vi "M9700 Modbus Demo.vi"(0 "Serial Port:":refnum<visa-resource-name>="COM1", 1 "Voltage(V)":sgl=10.0 format="%#.5g", 2 "Current(A)":sgl=1.0 format="%#.5g", 3 "Resistance(Ohm)":sgl=100.0 format="%#.5g", 4 "Power(W)":sgl=30.0 format="%#.5g", 5 "error in (no error)":errorcluster, 6 "BaudRate:":u16(ring)=1 items=["  2400", "  9600", "  14400", "  28800", "  57600", "  115200"], 7 "Set Voltage":bool, 10 "Load Address":u8=1 min=1 max=200 format="%.0x", 11 "Set Current":bool, 12 "Input ON":bool, 13 "Set Resistance":bool, 14 "Input OFF":bool, 15 "Set Power":bool, 16 "Read Actual Value":bool, 17 "Exit":bool, 18 "Read Input State":bool) -> (19 "error out":errorcluster)   [LabVIEW 2014]
uses:
  M9700 Driver/86/vi.lib/M9700 Modbus.llb/CTL CMD Register.ctl
  M9700 Driver/85/vi.lib/M9700 Modbus.llb/CTL Register Address.ctl
  <vilib>/Instr/_visa.llb/VISA Configure Serial Port (Instr).vi
panel:
  in  "Configure Serial Port":bool
  in  "Short Mode":bool
  out "Actual Power(W)":sgl format="%#.5g"
  out "Actual Resistance(Ohm)":sgl format="%#.5g"
  out "Actual Current(A)":sgl format="%#.5g"
  out "Actual Voltage(V)":sgl format="%#.5g"
  out "Input State":bool
  in  "About":bool
  in  "Parity:":u16(ring) items=["  None", "  Odd", "  Even"]
  # "This example shows how communication is generated between M97 series electronic load \n and LabVIEW Program by M9700 MODBUS LabVIEW Driver. \n."
  # "Serial Port Parameter:"
  # "Work Mode:"
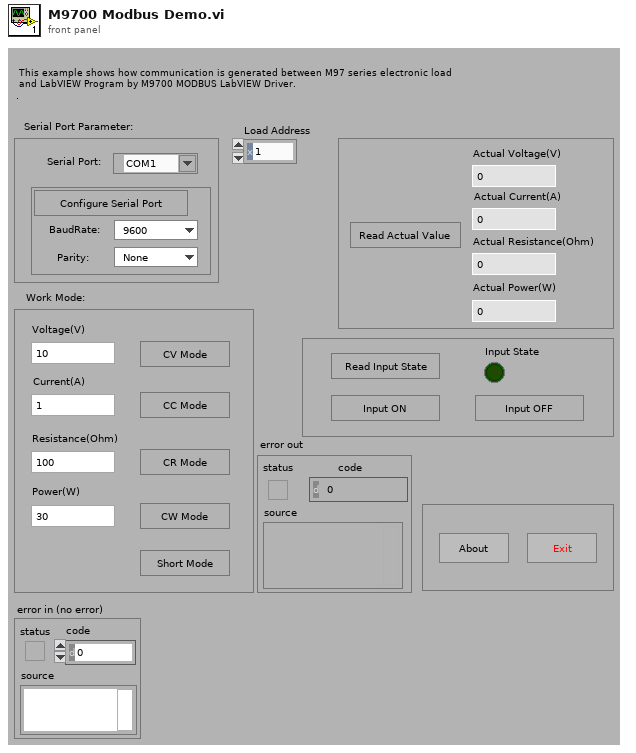
[diagram p1: front panel]
types:
  T1 = typedef "CTL CMD Register.ctl" = u8
  T2 = typedef "CTL Register Address.ctl" = u16
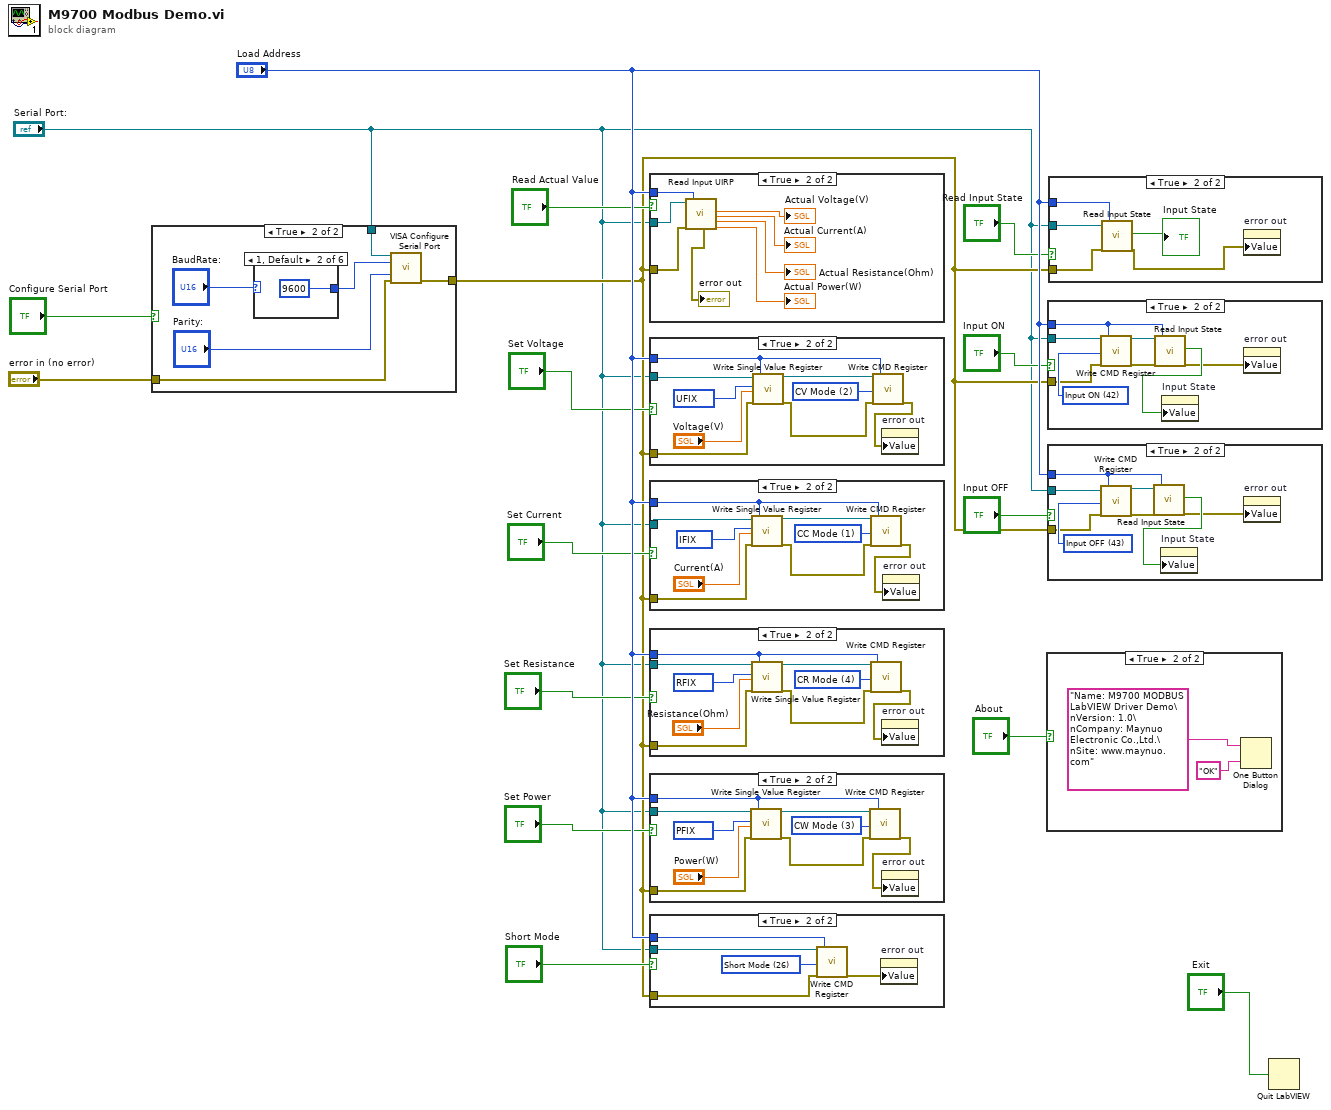
[diagram p0: block diagram]
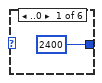
[diagram p3: hidden frame]
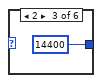
[diagram p4: hidden frame]
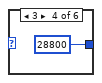
[diagram p5: hidden frame]
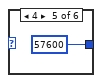
[diagram p6: hidden frame]
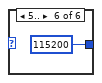
[diagram p7: hidden frame]
diagram:
  n1 = case shown="True" "Configure Serial Port" {
    tunnel: [w17 w23] -> w4
    tunnel: "Serial Port:" -> [_ w19]
    tunnel: "error in (no error)" -> [w17 w18]
    frame False {
    }
    frame True {
      n2 = case shown="1, Default" "BaudRate:" {
        tunnel: [2400 9600 14400 28800 57600 115200] -> w21
        frame ..0 {
        }
        frame 1, Default {
        }
        frame 2 {
        }
        frame 3 {
        }
        frame 4 {
        }
        frame 5.. {
        }
      }
      n3 = call-poly "VISA Configure Serial Port"("VISA resource name"=w19, "baud rate (9600)"=w21, "parity (0:none)"="Parity:", "error in (no error)"=w18) -> ("error out"=w23:errorcluster)  [unwired: 2 in, 9 out]
    }
  }
  n4 = case shown="True" "Read Actual Value" {
    tunnel: "Load Address" -> [_ w37]
    tunnel: "Serial Port:" -> [_ w36]
    tunnel: w4 -> [_ w31]
    frame False {
    }
    frame True {
      n5 = call "Read Input UIRP.vi"("VISA resource name"=w36, "error in"=w31, "Load Address"=w37) -> ("error out"=→"error out":errorcluster, "Actual Voltage(V)"=→"Actual Voltage(V)":sgl, "Actual Current(A)"=→"Actual Current(A)":sgl, "Actual Resistance(Ohm)"=→"Actual Resistance(Ohm)":sgl, "Actual Power(W)"=→"Actual Power(W)":sgl)  [unwired: 12 out]
    }
  }
  n6 = case shown="True" "Set Voltage" {
    tunnel: "Load Address" -> [_ w42]
    tunnel: "Serial Port:" -> [_ w46]
    tunnel: w4 -> [_ w40]
    frame False {
    }
    frame True {
      w41 = T1 2 items=["CC Mode"=1, "CV Mode"=2, "CW Mode"=3, "CR Mode"=4, "Short Mode"=26, "Set SysPara"=41, "Input ON"=42, "Input OFF"=43] ("CMD Register Value")
      w44 = T2 2563 items=["REMOTE"=1283, "ISTATE"=1296, "CMD"=2560, "IFIX"=2561, "UFIX"=2563, "PFIX"=2565, "RFIX"=2567, "IMAX"=2612, "UMAX"=2614, "PMAX"=2616, "U"=2816, "I"=2818, "MODEL"=2822, "EDITION"=2823] ("Register Address")
      n7 = call "Write Single Value Register.vi"("VISA resource name"=w46, "Starting Address(HEX)"=w44, "Register Single Value"="Voltage(V)", "error in"=w40, "Load Address"=w42) -> ("VISA resource name out"=w43:refnum<visa-resource-name>, "error out"=w39:errorcluster)  [unwired: 13 out]
      n8 = call "Write CMD Register.vi"("VISA resource name"=w43, "CMD Value"=w41, "error in"=w39, "Load Address"=w42) -> ("error out"=w38:errorcluster)  [unwired: 15 out]
      n9 = property on="error out" class="Clust (strict)"("Value"=w38) -> ()  [unwired: 2 in, 2 out]
    }
  }
  n10 = case shown="True" "Set Current" {
    tunnel: "Load Address" -> [_ w55]
    tunnel: "Serial Port:" -> [_ w51]
    tunnel: w4 -> [_ w49]
    frame False {
    }
    frame True {
      w52 = T1 1 items=["CC Mode"=1, "CV Mode"=2, "CW Mode"=3, "CR Mode"=4, "Short Mode"=26, "Set SysPara"=41, "Input ON"=42, "Input OFF"=43] ("CMD Register Value")
      w54 = T2 2561 items=["REMOTE"=1283, "ISTATE"=1296, "CMD"=2560, "IFIX"=2561, "UFIX"=2563, "PFIX"=2565, "RFIX"=2567, "IMAX"=2612, "UMAX"=2614, "PMAX"=2616, "U"=2816, "I"=2818, "MODEL"=2822, "EDITION"=2823] ("Register Address")
      n11 = call "Write Single Value Register.vi"("VISA resource name"=w51, "Starting Address(HEX)"=w54, "Register Single Value"="Current(A)", "error in"=w49, "Load Address"=w55) -> ("VISA resource name out"=w50:refnum<visa-resource-name>, "error out"=w48:errorcluster)  [unwired: 13 out]
      n12 = call "Write CMD Register.vi"("VISA resource name"=w50, "CMD Value"=w52, "error in"=w48, "Load Address"=w55) -> ("error out"=w47:errorcluster)  [unwired: 15 out]
      n13 = property on="error out" class="Clust (strict)"("Value"=w47) -> ()  [unwired: 2 in, 2 out]
    }
  }
  n14 = case shown="True" "Set Resistance" {
    tunnel: "Serial Port:" -> [_ w62]
    tunnel: "Load Address" -> [_ w64]
    tunnel: w4 -> [_ w58]
    frame False {
    }
    frame True {
      w59 = T1 4 items=["CC Mode"=1, "CV Mode"=2, "CW Mode"=3, "CR Mode"=4, "Short Mode"=26, "Set SysPara"=41, "Input ON"=42, "Input OFF"=43] ("CMD Register Value")
      w61 = T2 2567 items=["REMOTE"=1283, "ISTATE"=1296, "CMD"=2560, "IFIX"=2561, "UFIX"=2563, "PFIX"=2565, "RFIX"=2567, "IMAX"=2612, "UMAX"=2614, "PMAX"=2616, "U"=2816, "I"=2818, "MODEL"=2822, "EDITION"=2823] ("Register Address")
      n15 = call "Write Single Value Register.vi"("VISA resource name"=w62, "Starting Address(HEX)"=w61, "Register Single Value"="Resistance(Ohm)", "error in"=w58, "Load Address"=w64) -> ("VISA resource name out"=w63:refnum<visa-resource-name>, "error out"=w57:errorcluster)  [unwired: 13 out]
      n16 = call "Write CMD Register.vi"("VISA resource name"=w63, "CMD Value"=w59, "error in"=w57, "Load Address"=w64) -> ("error out"=w56:errorcluster)  [unwired: 15 out]
      n17 = property on="error out" class="Clust (strict)"("Value"=w56) -> ()  [unwired: 2 in, 2 out]
    }
  }
  n18 = case shown="True" "Set Power" {
    tunnel: "Serial Port:" -> [_ w73]
    tunnel: "Load Address" -> [_ w71]
    tunnel: w4 -> [_ w68]
    frame False {
    }
    frame True {
      w69 = T1 3 items=["CC Mode"=1, "CV Mode"=2, "CW Mode"=3, "CR Mode"=4, "Short Mode"=26, "Set SysPara"=41, "Input ON"=42, "Input OFF"=43] ("CMD Register Value")
      w70 = T2 2565 items=["REMOTE"=1283, "ISTATE"=1296, "CMD"=2560, "IFIX"=2561, "UFIX"=2563, "PFIX"=2565, "RFIX"=2567, "IMAX"=2612, "UMAX"=2614, "PMAX"=2616, "U"=2816, "I"=2818, "MODEL"=2822, "EDITION"=2823] ("Register Address")
      n19 = call "Write Single Value Register.vi"("VISA resource name"=w73, "Starting Address(HEX)"=w70, "Register Single Value"="Power(W)", "error in"=w68, "Load Address"=w71) -> ("VISA resource name out"=w72:refnum<visa-resource-name>, "error out"=w66:errorcluster)  [unwired: 13 out]
      n20 = call "Write CMD Register.vi"("VISA resource name"=w72, "CMD Value"=w69, "error in"=w66, "Load Address"=w71) -> ("error out"=w65:errorcluster)  [unwired: 15 out]
      n21 = property on="error out" class="Clust (strict)"("Value"=w65) -> ()  [unwired: 2 in, 2 out]
    }
  }
  n22 = case shown="True" "Short Mode" {
    tunnel: "Serial Port:" -> [_ w78]
    tunnel: "Load Address" -> [_ w76]
    tunnel: w4 -> [_ w75]
    frame False {
    }
    frame True {
      w77 = T1 26 items=["CC Mode"=1, "CV Mode"=2, "CW Mode"=3, "CR Mode"=4, "Short Mode"=26, "Set SysPara"=41, "Input ON"=42, "Input OFF"=43] ("CMD Register Value")
      n23 = call "Write CMD Register.vi"("VISA resource name"=w78, "CMD Value"=w77, "error in"=w75, "Load Address"=w76) -> ("error out"=w74:errorcluster)  [unwired: 15 out]
      n24 = property on="error out" class="Clust (strict)"("Value"=w74) -> ()  [unwired: 2 in, 2 out]
    }
  }
  n25 = case shown="True" "About" {
    frame False {
    }
    frame True {
      n26 = One Button Dialog(message="Name: M9700 MODBUS LabVIEW Driver Demo\nVersion: 1.0\nCompany: Maynuo Electronic Co.,Ltd.\nSite: www.maynuo.com", button name ("OK")="OK") -> ()  [unwired: 1 out]
    }
  }
  n27 = case shown="True" "Input ON" {
    tunnel: "Serial Port:" -> [_ w88]
    tunnel: "Load Address" -> [_ w84]
    tunnel: w4 -> [_ w83]
    frame False {
    }
    frame True {
      w87 = T1 42 items=["CC Mode"=1, "CV Mode"=2, "CW Mode"=3, "CR Mode"=4, "Short Mode"=26, "Set SysPara"=41, "Input ON"=42, "Input OFF"=43] ("CMD Register Value")
      n28 = call "Write CMD Register.vi"("VISA resource name"=w88, "CMD Value"=w87, "error in"=w83, "Load Address"=w84) -> ("VISA resource name out"=w86:refnum<visa-resource-name>, "error out"=w82:errorcluster)  [unwired: 14 out]
      n29 = call "Read Input State.vi"("VISA resource name"=w86, "error in"=w82, "Load Address"=w84) -> ("Input State(ON/OFF)"=w85:bool, "error out"=w81:errorcluster)  [unwired: 15 out]
      n30 = property on="Input State" class="Bool (strict)"("Value"=w85) -> ()  [unwired: 2 in, 2 out]
      n31 = property on="error out" class="Clust (strict)"("Value"=w81) -> ()  [unwired: 2 in, 2 out]
    }
  }
  n32 = case shown="True" "Input OFF" {
    tunnel: "Serial Port:" -> [_ w96]
    tunnel: "Load Address" -> [_ w93]
    tunnel: w4 -> [_ w91]
    frame False {
    }
    frame True {
      w95 = T1 43 items=["CC Mode"=1, "CV Mode"=2, "CW Mode"=3, "CR Mode"=4, "Short Mode"=26, "Set SysPara"=41, "Input ON"=42, "Input OFF"=43] ("CMD Register Value")
      n33 = call "Write CMD Register.vi"("VISA resource name"=w96, "CMD Value"=w95, "error in"=w91, "Load Address"=w93) -> ("VISA resource name out"=w94:refnum<visa-resource-name>, "error out"=w90:errorcluster)  [unwired: 14 out]
      n34 = call "Read Input State.vi"("VISA resource name"=w94, "error in"=w90, "Load Address"=w93) -> ("Input State(ON/OFF)"=w92:bool, "error out"=w89:errorcluster)  [unwired: 15 out]
      n35 = property on="Input State" class="Bool (strict)"("Value"=w92) -> ()  [unwired: 2 in, 2 out]
      n36 = property on="error out" class="Clust (strict)"("Value"=w89) -> ()  [unwired: 2 in, 2 out]
    }
  }
  n37 = case shown="True" "Read Input State" {
    tunnel: "Load Address" -> [_ w101]
    tunnel: "Serial Port:" -> [_ w99]
    tunnel: w4 -> [_ w98]
    frame False {
    }
    frame True {
      n38 = call "Read Input State.vi"("VISA resource name"=w99, "error in"=w98, "Load Address"=w101) -> ("Input State(ON/OFF)"=→"Input State":bool, "error out"=w97:errorcluster)  [unwired: 15 out]
      n39 = property on="error out" class="Clust (strict)"("Value"=w97) -> ()  [unwired: 2 in, 2 out]
    }
  }
  n40 = Quit LabVIEW(quit? (T)="Exit") -> ()
